vi "Create Session.vi"(7 "option string":string, 8 "error in":errorcluster, 9 "reset":bool, 11 "session reservation in":refnum<class "Session Reservation.lvclass">) -> (0 "error out":errorcluster, 1 "channel lists":string, 2 "sessions":refnum<k15>, 3 "session reservation out":refnum<class "Session Reservation.lvclass">)   [LabVIEW 2020, in "MeasurementLink niDCPower.lvlib"]
uses:
  MeasurementLink Session Management/Session Reservation/Session Reservation.lvclass
  MeasurementLink Session Management/Session Reservation/Session Reservation.lvclass/Session Reservation.ctl
  MeasurementLink Session Management/Session Reservation/Create Sessions Impl.vi
  Instrument/Instrument.lvclass
  \\tsclient\C/dev/measurementlink-labview/Source/Runtime/MeasurementLink Instrument/IInstrument/IInstrument.lvclass
  MeasurementLink gRPC Utilities/Service Location FGV.vi
  MeasurementLink Instrument/IInstrument/IInstrument.lvclass
  MeasurementLink niDCPower.lvlib
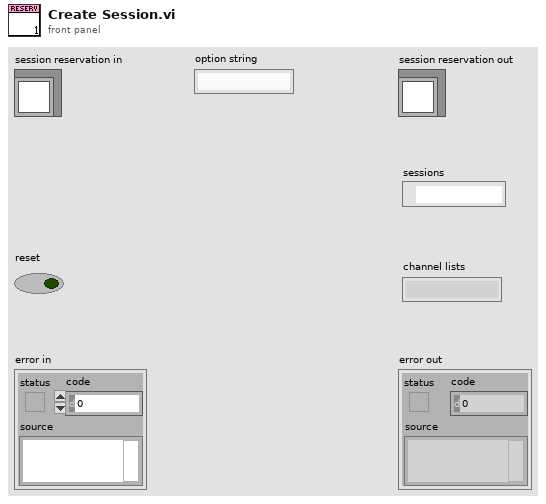
[diagram p1: front panel]
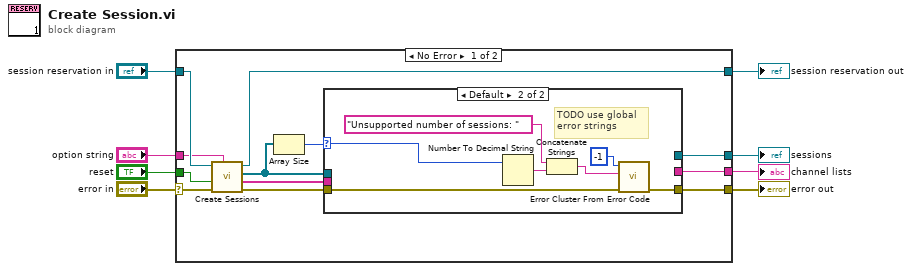
[diagram p0: block diagram]
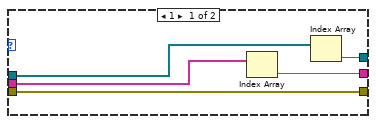
[diagram p2: hidden frame]
diagram:
  n1 = case shown="No Error" "error in" {
    selector: "error in" -> [w18 w34]
    tunnel: [w9 w34] -> w7
    tunnel: [w19 w33] -> w5
    tunnel: "session reservation in" -> [w20 w33]
    tunnel: "option string" -> [w16 _]
    tunnel: "reset" -> [w17 _]
    tunnel: [w13 _] -> w2
    tunnel: [w11 _] -> w1
    frame No Error {
      n2 = call "Create Sessions.vi"("option string"=w16, "error in"=w18, "reset"=w17, "session reservation in"=w20) -> ("error out"=w10:errorcluster, "channel lists"=w12:string[], "sessions"=w14:refnum<k15>[], "session reservation out"=w19:refnum<class "Session Reservation.lvclass">)  [unwired: 4 in]
      n3 = Array Size(array=w14) -> (size(s)=w15:i32)
      n4 = case shown="Default" w15 {
        selector: w15 -> [_ w28]
        tunnel: [w21 w31] -> w9
        tunnel: w14 -> [w24 _]
        tunnel: [w25 _] -> w13
        tunnel: w12 -> [w23 _]
        tunnel: [w22 _] -> w11
        tunnel: w10 -> [w21 w26]
        frame 1 {
          n5 = Index Array(array=w23) -> (element=w22:string)  [unwired: 1 in]
          n6 = Index Array(array=w24) -> (element=w25:refnum<k15>)  [unwired: 1 in]
        }
        frame Default {
          # "TODO use global\nerror strings"
          n7 = Number To Decimal String(number=w28) -> (decimal integer string=w29:string)  [unwired: 1 in]
          n8 = Concatenate Strings("Unsupported number of sessions: " ("error message (\"\")"), w29) -> (w27:string)
          n9 = call <vilib>:"Error Cluster From Error Code.vi"("error in (no error)"=w26, "error message (\"\")"=w27, "error code (0)"=-1) -> ("error out"=w31:errorcluster)  [unwired: 6 in]
        }
      }
    }
    frame Error {
    }
  }
  "error out" <- w7
  "session reservation out" <- w5
  "sessions" <- w2
  "channel lists" <- w1
